vi "Start Module.vi"(8 "error in":errorcluster, 11 "Run as Singleton? (F)":bool) -> (0 "error out":errorcluster, 1 "Wait for Event Sync?":bool, 2 "FGen Broadcast Events":T1, 3 "Module ID":i32)   [LabVIEW 2020, in "FGen.lvlib"]
doc: "Launches an instance of the module Main VI. After calling this VI, you can optionally register for broadcast events from the module by wiring the broadcast events output of this VI to a <b>Register For Events</b> function. \n\nAfter the optional Register For Events function call, you should always call the <b>Synchronize Module Events.vi</b> for this module with the 'Wait for Event Sync?' output of this VI to the corresponding input of the Synchronize Module Events.vi. \n\nTo see an example of the proper wiring pattern, see the \"Run New Module: Value Change\" event frame in the API Tester VI for this module.\n_____\nBased on DQMH Project Template 6.0.0.91."
uses:
  FGen.lvlib
  Broadcast Events--cluster.ctl
  Did Init Argument--cluster.ctl
  Status Updated Argument--cluster.ctl
  Error Reported Argument--cluster.ctl
  Stop Argument--cluster.ctl
  Get Module Execution Status Argument--cluster.ctl
  Oscilloscope Lista Argument--cluster.ctl
  Module Running State--enum.ctl
  <vilib>/Delacor/Delacor QMH/Libraries/Cloneable Module Admin_class/Delacor_lib_QMH_Cloneable Module Admin.lvclass
  C:/Program Files (x86)/National Instruments/LabVIEW 2020/vi.lib/Delacor/Delacor QMH/Libraries/Module Admin_class/Delacor_lib_QMH_Module Admin.lvclass
  VI Reference Management/Main VI Type--strict_vi_ref.ctl
  <vilib>/Delacor/Delacor QMH/Libraries/Cloneable Module Admin_class/Delacor_lib_QMH_Cloneable Module Admin.lvclass/Delacor_lib_QMH_Cloneable Module Admin.ctl
  <vilib>/Delacor/Delacor QMH/Libraries/Module Admin_class/Delacor_lib_QMH_Module Admin.lvclass/Delacor_lib_QMH_Module Admin.ctl
  <vilib>/Delacor/Delacor QMH/Libraries/Cloneable Module Admin_class/Delacor_lib_QMH_Set Module ID.vi
  <vilib>/Delacor/Delacor QMH/Libraries/Module Admin_class/Delacor_lib_QMH_Set External Launch.vi
  Main.vi
  <vilib>/Utility/error.llb/Error Cluster From Error Code.vi
  <vilib>/ErrorRing/Error Ring.xnode
  Clone Registration/Clone Registration.lvlib
  VI Reference Management/VI Reference Management.lvlib
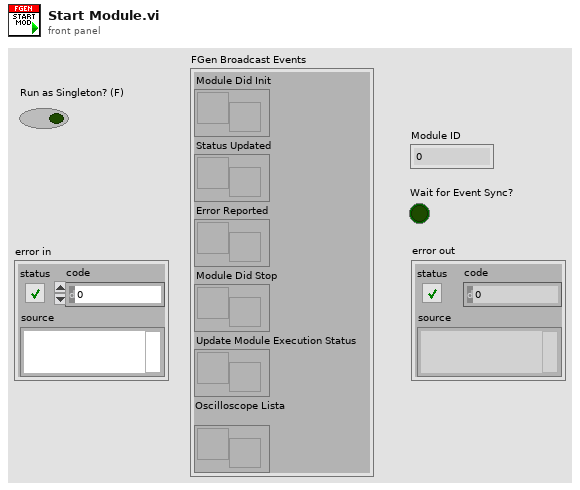
[diagram p1: front panel]
types:
  T1 = typedef "FGen.lvlib/Broadcast Events--cluster.ctl" = cluster{"Module Did Init":refnum<user-event>, "Status Updated":refnum<user-event>, "Error Reported":refnum<user-event>, "Module Did Stop":refnum<user-event>, "Update Module Execution Status":refnum<user-event>, "Oscilloscope Lista":refnum<user-event>}
  T2 = typedef "FGen.lvlib/Module Running State--enum.ctl" = enum16{"Not Running", "Running as Cloneable", "Running as Singleton"}
  T3 = enum32{"Bad", "Idle", "Run top level", "Running"}
  T4 = typedef "FGen.lvlib/VI Reference Management.lvlib/Main VI Type--strict_vi_ref.ctl" = refnum<vi>
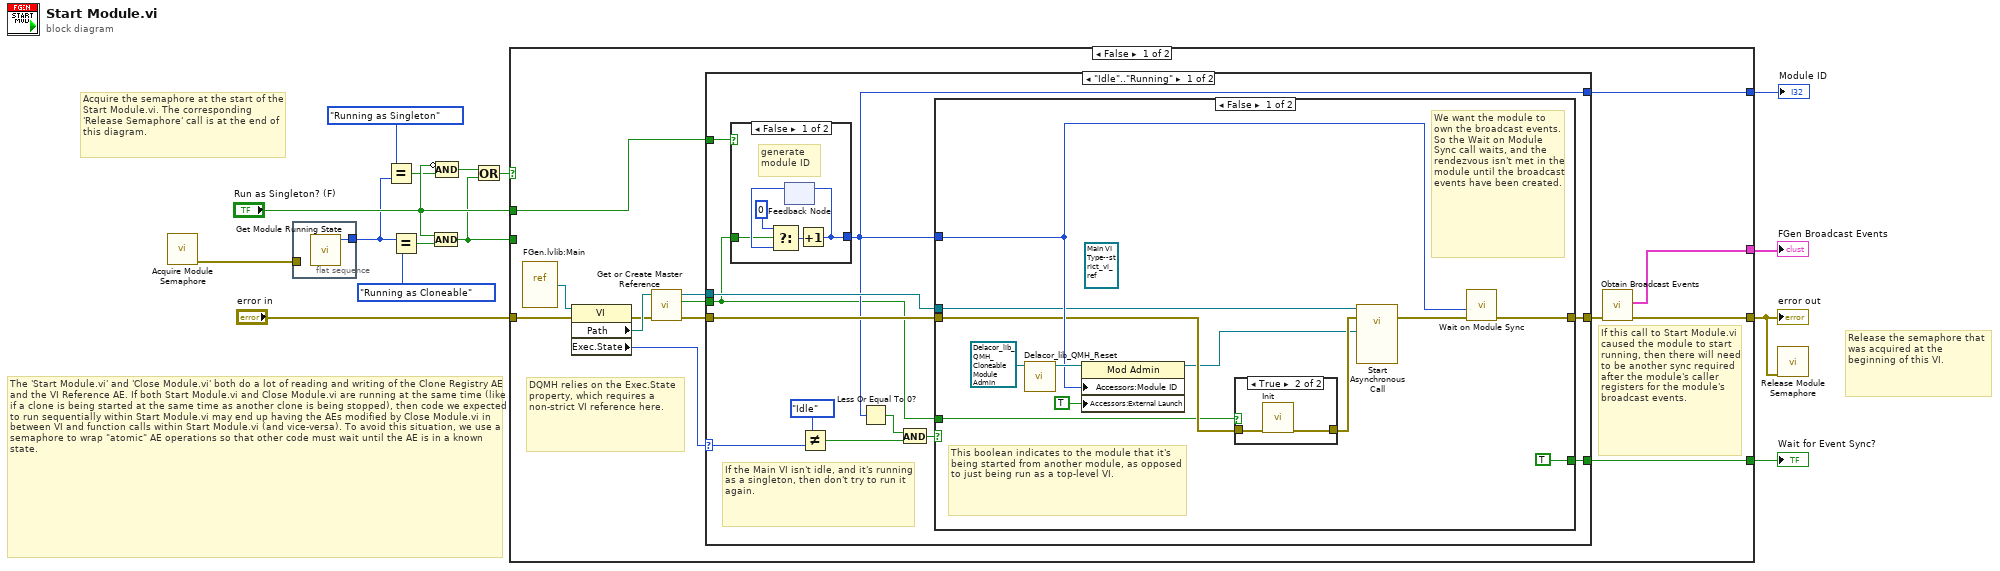
[diagram p0: block diagram]
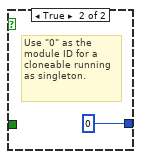
[diagram p2: hidden frame]
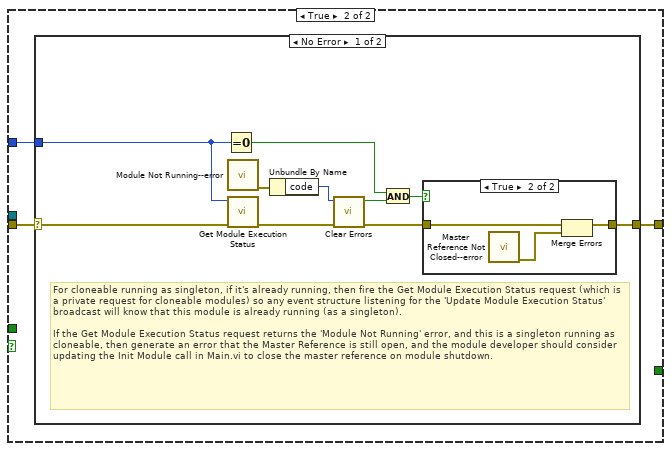
[diagram p4: hidden frame]
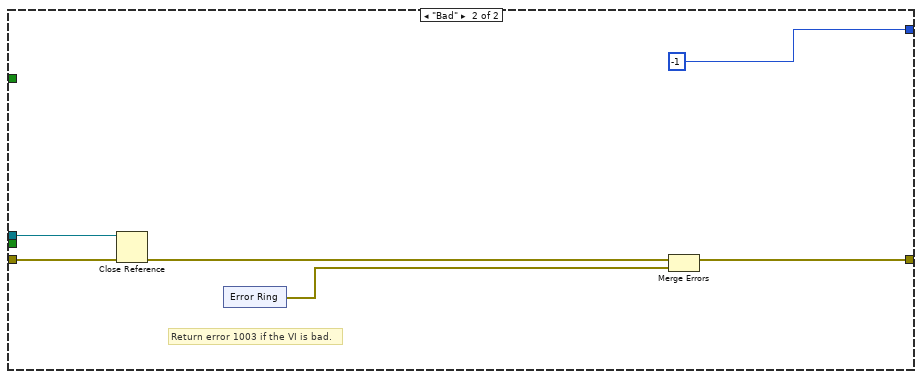
[diagram p7: hidden frame]
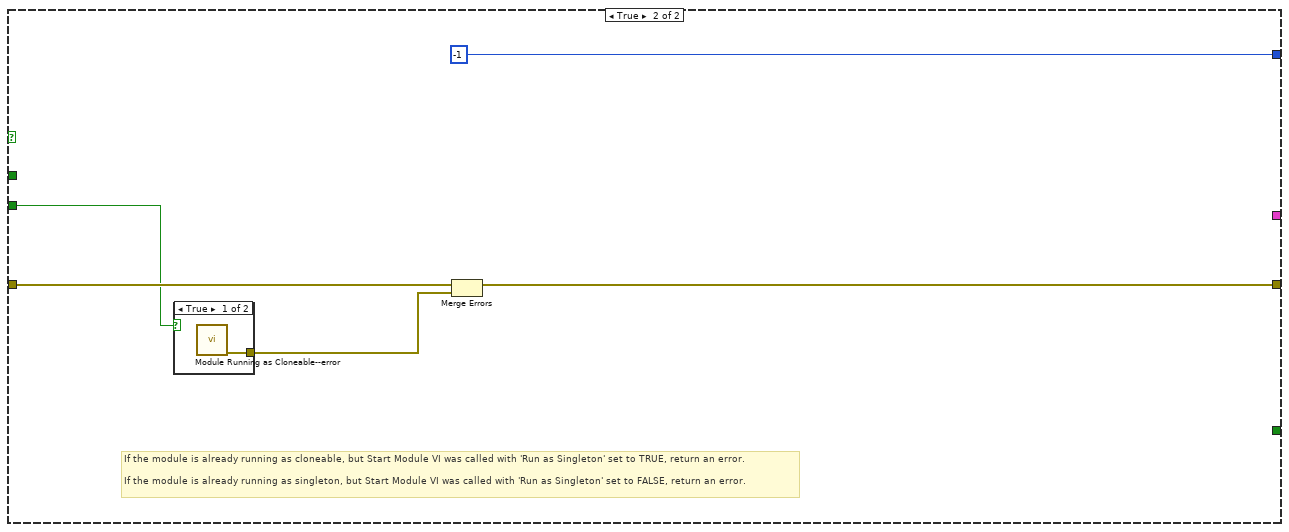
[diagram p8: hidden frame]
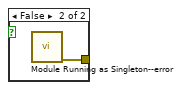
[diagram p9: hidden frame]
diagram:
  # "Release the semaphore that was acquired at the beginning of this VI."
  # "The 'Start Module.vi' and 'Close Module.vi' both do a lot of reading and writing of the Clone Registry AE and the VI Reference AE. If both Start Module.vi and Close Module.vi are running at the same time (like if a clone is being started at the same time as another clone is being stopped), then code we expected to run sequentially within Start Module.vi may end up having the AEs modified by Close Module.vi in between VI and function calls within Start Module.vi (and vice-versa). To avoid this situation, we use a semaphore to wrap \"atomic\" AE operations so that other code must wait until the AE is in a known state."
  # "Acquire the semaphore at the start of the Start Module.vi. The corresponding 'Release Semaphore' call is at the end of this diagram."
  n1 = call "Acquire Module Semaphore.vi"() -> ("error out"=w2:errorcluster)  [unwired: 11 in]
  n2 = flat-sequence {
    tunnel: [w16] -> w5
    tunnel: w2 -> [_]
    frame #0 {
      n3 = call "Get Module Running State.vi"() -> ("Module Running State"=w16:T2)  [unwired: 11 in]
    }
  }
  n4 = Equal?(x=Module_Running_State--enum."Running as Singleton", y=w5) -> (x = y?=w6:bool)
  n5 = Equal?(x=w5, y=Module_Running_State--enum."Running as Cloneable") -> (x = y?=w10:bool)
  n6 = And(x="Run as Singleton? (F)", y=w10) -> (x .and. y?=w3:bool)
  n7 = Compound Arithmetic op=AND(invert "Run as Singleton? (F)", w6) -> (w8:bool)
  n8 = Or(x=w8, y=w3) -> (x .or. y?=w9:bool)
  n9 = case shown="False" w9 {
    tunnel: "error in" -> [w30 w96]
    tunnel: [w28 w95] -> w1
    tunnel: [w27 _] -> w14
    tunnel: [w26 _] -> w13
    tunnel: [w22 -1] -> w12
    tunnel: "Run as Singleton? (F)" -> [w18 _]
    tunnel: w3 -> [_ w92]
    frame False {
      # "DQMH relies on the Exec.State property, which requires a non-strict VI reference here."
      # "If this call to Start Module.vi caused the module to start running, then there will need to be another sync required after the module's caller registers for the module's broadcast events."
      n10 = vi-ref "FGen.lvlib:Main.vi"() -> (w21:refnum<vi>)
      n11 = property class="VI"(reference=w21, error in=w30) -> (error out=w24:errorcluster, "Path"=w25:path, "Exec.State"=w19:T3)  [unwired: 1 out]
      n12 = call "Get or Create Master Reference.vi"("error in (no error)"=w24, "Main VI Path"=w25) -> ("error out"=w23:errorcluster, "New Reference Created"=w17:bool, "Master Reference"=w20:T4)  [unwired: 7 in]
      n13 = case shown="\"Idle\"..\"Running\"" w19 {
        selector: w19 -> [w38 _]
        tunnel: w23 -> [w42 w87]
        tunnel: w20 -> [w40 w86]
        tunnel: [w39 w84] -> w29
        tunnel: [w41 _] -> w26
        tunnel: [w33 -1] -> w22
        tunnel: w18 -> [w32 _]
        tunnel: w17 -> [w31 _]
        frame "Idle".."Running" {
          # "If the Main VI isn't idle, and it's running as a singleton, then don't try to run it again."
          n14 = case shown="False" w32 {
            tunnel: [w47 0] -> w33
            tunnel: w31 -> [w43 _]
            frame False {
              # "generate module ID"
              n15 = feedback #1() -> (w45:i32)  [unwired: 1 in]
              n16 = Select(t=0, s=w43, f=w45) -> (s? t:f=w46:i32)
              n17 = Increment(x=w46) -> (x+1=w47:i32)
              n18 = feedback-in #1(w47) -> ()
            }
            frame True {
              # "Use \"0\" as the module ID for a cloneable running as singleton."
            }
          }
          n19 = Not Equal?(x=T3."Idle", y=w38) -> (x != y?=w36:bool)
          n20 = Less Or Equal To 0?(x=w33) -> (x <= 0?=w34:bool)
          n21 = And(x=w34, y=w36) -> (x .and. y?=w35:bool)
          n22 = case shown="False" w35 {
            tunnel: w42 -> [w52 w65]
            tunnel: [TRUE _] -> w41
            tunnel: w40 -> [w51 _]
            tunnel: [w55 w64] -> w39
            tunnel: w33 -> [w56 w66]
            tunnel: w31 -> [w49 _]
            frame False {
              (unwired) T4 refnum ("Main VI Type")
              # "We want the module to own the broadcast events. So the Wait on Module Sync call waits, and the rendezvous isn't met in the module until the broadcast events have been created."
              # "This boolean indicates to the module that it's being started from another module, as opposed to just being run as a top-level VI."
              n23 = call-dynamic "Delacor_lib_QMH_Reset.vi"("Mod Admin in"=refnum<class "Delacor_lib_QMH_Cloneable Module Admin.lvclass"> refnum) -> ("Mod Admin out"=w59:refnum<class "Delacor_lib_QMH_Cloneable Module Admin.lvclass">)  [unwired: 9 in, 1 out]
              n24 = property class="Mod Admin"(reference=w59, "Accessors:Module ID"=w56, "Accessors:External Launch"=TRUE) -> (reference out=w50:refnum<class "Delacor_lib_QMH_Cloneable Module Admin.lvclass">)  [unwired: 1 in, 1 out]
              n25 = case shown="True" w49 {
                tunnel: [w61 w63] -> w53
                tunnel: w52 -> [w61 w62]
                frame False {
                }
                frame True {
                  n26 = call "Init.vi"("error in (no error)"=w62) -> ("error out"=w63:errorcluster)  [unwired: 7 in, 3 out]
                }
              }
              n27 = call-by-ref "Start Asynchronous Call"(reference=w51, error in=w53, "Module Admin"=w50) -> (error out=w54:errorcluster)  [unwired: 11 in, 1 out]
              n28 = call "Wait on Module Sync.vi"("error in"=w54, "Module ID"=w56) -> ("error out"=w55:errorcluster)  [unwired: 9 in]
            }
            frame True {
              n29 = case shown="No Error" w65 {
                selector: w65 -> [w76 w81]
                tunnel: w66 -> [w74 _]
                tunnel: [w67 w81] -> w64
                frame No Error {
                  # "For cloneable running as singleton, if it's already running, then fire the Get Module Execution Status request (which is a private request for cloneable modules) so any event structure listening for the 'Update Module Execution Status' broadcast will know that this module is already running (as a singleton).\n\nIf the Get Module Execution Status request returns the 'Module Not Running' error, and this is a singleton running as cloneable, then generate an error that the Master Reference is still open, and the module developer should consider updating the Init Module call in Main.vi to close the master reference on module shutdown."
                  n30 = Equal To 0?(x=w74) -> (x = 0?=w70:bool)
                  n31 = call "Module Not Running--error.vi"() -> ("error out"=w73:errorcluster)  [unwired: 11 in]
                  n32 = call "Get Module Execution Status.vi"("error in (no error)"=w76, "Module ID"=w74) -> ("error out"=w75:errorcluster)  [unwired: 9 in]
                  n33 = Unbundle By Name(w73) -> ("code"=w72:i32)
                  n34 = call <vilib>:"Clear Errors.vi"("error in (no error)"=w75, "specific error code to clear (0: all)"=w72) -> ("error out"=w69:errorcluster, "specific error cleared?"=w71:bool)  [unwired: 4 in]
                  n35 = And(x=w70, y=w71) -> (x .and. y?=w68:bool)
                  n36 = case shown="True" w68 {
                    tunnel: w69 -> [w77 w80]
                    tunnel: [w77 w78] -> w67
                    frame False {
                    }
                    frame True {
                      n37 = call "Master Reference Not Closed--error.vi"() -> ("error out"=w79:errorcluster)  [unwired: 11 in]
                      n38 = Merge Errors(w80, w79) -> (w78:errorcluster)
                    }
                  }
                }
                frame Error {
                }
              }
            }
          }
        }
        frame "Bad" {
          # "Return error 1003 if the VI is bad."
          n39 = Close Reference(reference=w86, error in (no error)=w87) -> (error out=w85:errorcluster)
          n40 = xnode "Error Ring"() -> ("error out"=w83:errorcluster)
          n41 = Merge Errors(w85, w83) -> (w84:errorcluster)
        }
      }
      n42 = call "Obtain Broadcast Events.vi"("error in (no error)"=w29) -> ("error out"=w28:errorcluster, "FGen Broadcast Events"=w27:T1)  [unwired: 9 in]
    }
    frame True {
      # "If the module is already running as cloneable, but Start Module VI was called with 'Run as Singleton' set to TRUE, return an error.\n\nIf the module is already running as singleton, but Start Module VI was called with 'Run as Singleton' set to FALSE, return an error."
      n43 = case shown="True" w92 {
        tunnel: [w97 w98] -> w93
        frame True {
          n44 = call "Module Running as Cloneable--error.vi"() -> ("error out"=w97:errorcluster)  [unwired: 11 in]
        }
        frame False {
          n45 = call "Module Running as Singleton--error.vi"() -> ("error out"=w98:errorcluster)  [unwired: 11 in]
        }
      }
      n46 = Merge Errors(w96, w93) -> (w95:errorcluster)
    }
  }
  "error out" <- w1
  "FGen Broadcast Events" <- w14
  "Wait for Event Sync?" <- w13
  "Module ID" <- w12
  n47 = call "Release Module Semaphore.vi"("error in"=w1) -> ()  [unwired: 10 in, 1 out]
